vi "Three Pins Logic Gate Template.vi"(1 "Pin2":bool, 2 "Pin1":bool, 3 "Pin0":bool) -> (0 "Output":bool)   [LabVIEW 2012]
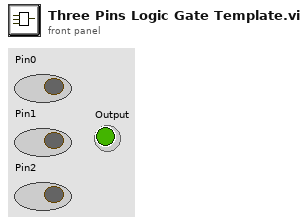
[diagram p1: front panel]
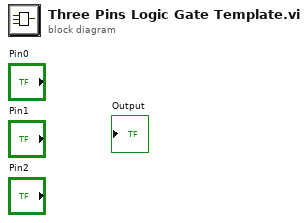
[diagram p0: block diagram]
diagram:
